vi "Write First Element.vi"(10 "First Element":refnum<k20>, 11 "XML Handler in":refnum<class "XML Handler.lvclass">) -> (3 "XML Handler out":refnum<class "XML Handler.lvclass">)   [LabVIEW 2020, in "XML Handler.lvclass"]
uses:
  XML Handler.lvclass
  XML Handler.lvclass/XML Handler.ctl
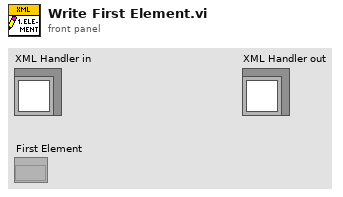
[diagram p1: front panel]
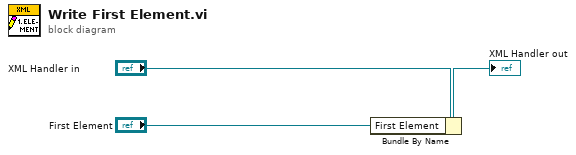
[diagram p0: block diagram]
diagram:
  n1 = Bundle By Name(cluster="XML Handler in", "First Element"="First Element") -> (→"XML Handler out":refnum<class "XML Handler.lvclass">)
